vi "Write RGB.vi"(8 "error in (no error)":errorcluster, 10 "Color Box":u32(colorbox), 11 "RGB in":refnum<class "RGB I2C.lvclass">) -> (0 "error out":errorcluster, 3 "RGB out":refnum<class "RGB I2C.lvclass">)   [LabVIEW 2020, in "CTI-Peripheral.lvlib" / "RGB I2C.lvclass"]
uses:
  RGB I2C.lvclass
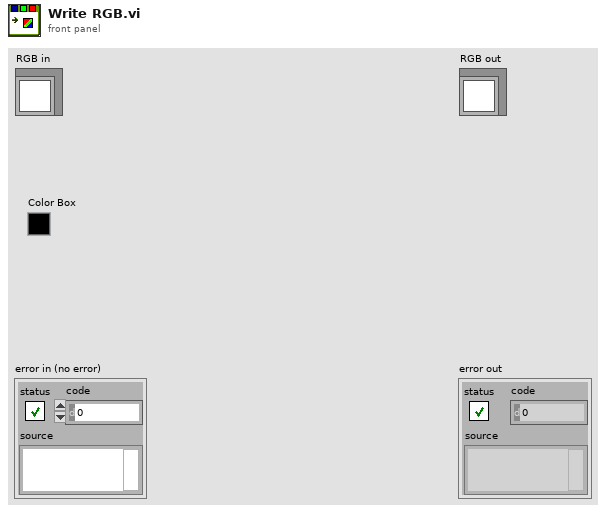
[diagram p1: front panel]
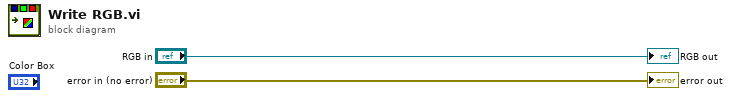
[diagram p0: block diagram]
diagram:
  "error out" <- "error in (no error)"
  "RGB out" <- "RGB in"
